vi "10 Balls.vi"() -> ()   [LabVIEW 2019]
uses:
  Team Code/TurretMode.ctl
  Team Code/MotorsGlobal.vi
  Team Code/JoysticksGlobal.vi
  Default10BallEnum.ctl
panel:
  in  "Delay After CurvaDir3":i32
  in  "RangeCurvaDir3":cluster{"output high":dbl, "output low":dbl}={"output high"=0.6, "output low"=-0.6} {"output low" format="%.2f"; "output high" format="%.2f"}
  in  "GainsCurvaDir3":T1={"proportional gain (Kc)"=1.0, "integral time (Ti, min)"=0.01, "derivative time (Td, min)"=0.0} {"derivative time (Td, min)" format="%.3f"; "integral time (Ti, min)" format="%.3f"; "proportional gain (Kc)" format="%.3f"}
  in  "Setpoint_CurvaDir3":dbl
  in  "TimeLimit_CurvaDir3":dbl
  in  "Delay After CurvaEsq2":i32
  in  "Delay After CurvaEsq1":i32
  in  "TimeLimit_Anda2":dbl
  in  "DelayAnda2":i32=300
  in  "Distance2":dbl
  in  "PID 10 Ball":T2(tab)
  in  "Distance1":dbl
  in  "DelayAnda1":i32=300
  in  "TimeLimit_Anda1":dbl
  in  "GainsCurvaEsq1":T1={"proportional gain (Kc)"=1.0, "integral time (Ti, min)"=0.01, "derivative time (Td, min)"=0.0} {"derivative time (Td, min)" format="%.3f"; "integral time (Ti, min)" format="%.3f"; "proportional gain (Kc)" format="%.3f"}
  in  "RangeCurvaEsq1":cluster{"output high":dbl, "output low":dbl}={"output high"=0.6, "output low"=-0.6} {"output low" format="%.2f"; "output high" format="%.2f"}
  in  "TimeLimit_CurvaEsq1":dbl
  in  "Setpoint_CurvaEsq1":dbl
  in  "Distance2":dbl
  in  "DelayAnda2":i32=300
  in  "TimeLimit_Anda2":dbl
  in  "GainsCurvaEsq2":T1={"proportional gain (Kc)"=1.0, "integral time (Ti, min)"=0.01, "derivative time (Td, min)"=0.0} {"derivative time (Td, min)" format="%.3f"; "integral time (Ti, min)" format="%.3f"; "proportional gain (Kc)" format="%.3f"}
  in  "RangeCurvaEsq2":cluster{"output high":dbl, "output low":dbl}={"output high"=0.6, "output low"=-0.6} {"output low" format="%.2f"; "output high" format="%.2f"}
  in  "TimeLimit_CurvaEsq2":dbl
  in  "Setpoint_CurvaEsq2":dbl
  in  "TimeLimit_AlinhaLL1":dbl
  in  "TimeLimit_Atira1":dbl
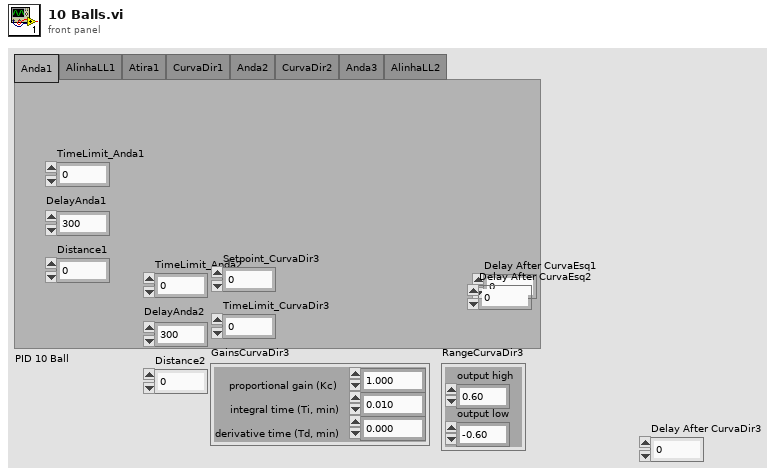
[diagram p1: front panel]
types:
  T1 = cluster{"proportional gain (Kc)":dbl, "integral time (Ti, min)":dbl, "derivative time (Td, min)":dbl}
  T2 = enum32{"Anda1", "AlinhaLL1", "Atira1", "CurvaDir1", "Anda2", "CurvaDir2", "Anda3", "AlinhaLL2"}
  T3 = typedef "Default10BallEnum.ctl" = enum16{"Reset1", "Anda1", "Reset2", "AndaAtras2", "CurvaEsq1", "Reset3", "Anda3", "CurvaEsq2", "Reset4", "AlinhaLL1", "Atira1", "CurvaDir3", "Reset5", "Anda4", "CurvaDir4", "Reset6", "Anda5", "AlinhaLL2", "Atira2"}
  T4 = typedef "TurretMode.ctl" = enum16{"Static", "Manual", "Automatic"}
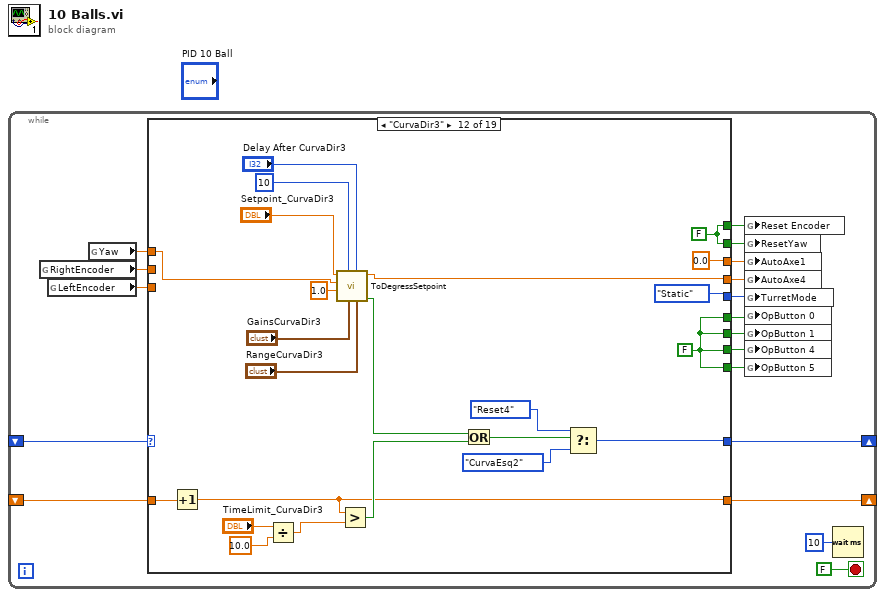
[diagram p0: block diagram]
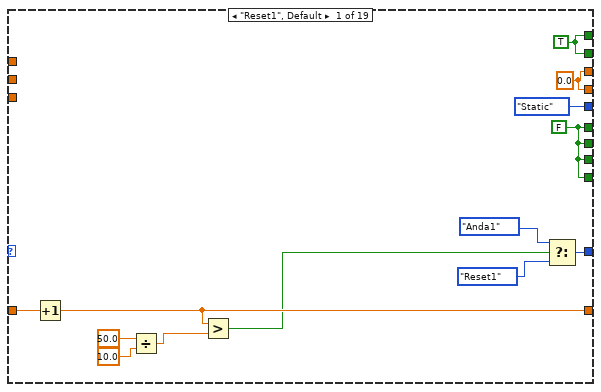
[diagram p2: hidden frame]
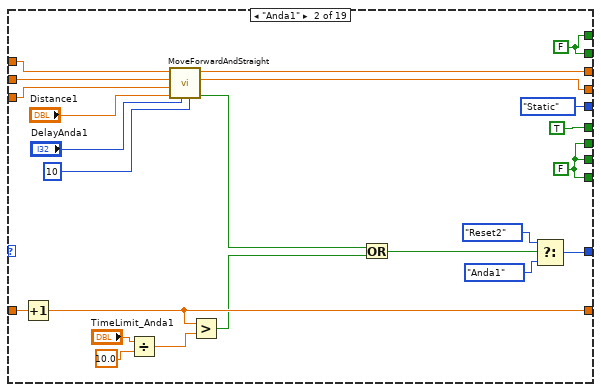
[diagram p3: hidden frame]
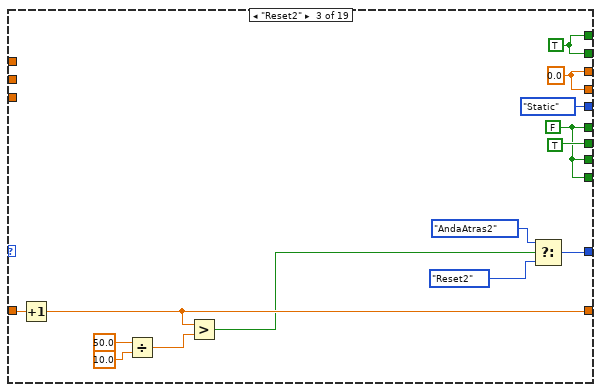
[diagram p4: hidden frame]
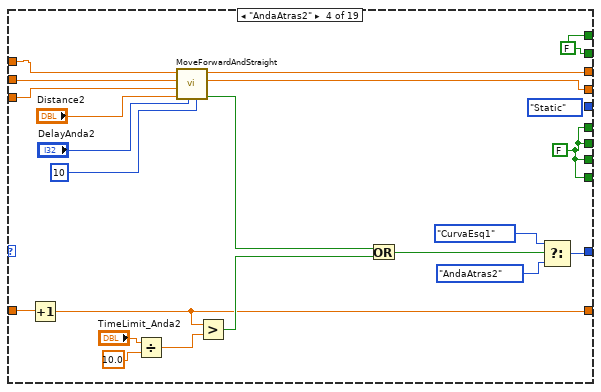
[diagram p5: hidden frame]
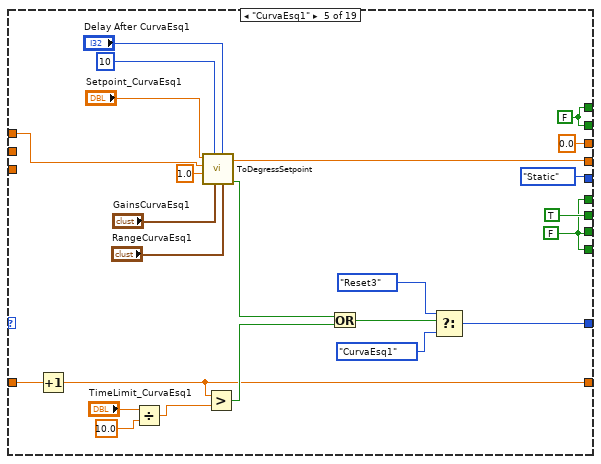
[diagram p6: hidden frame]
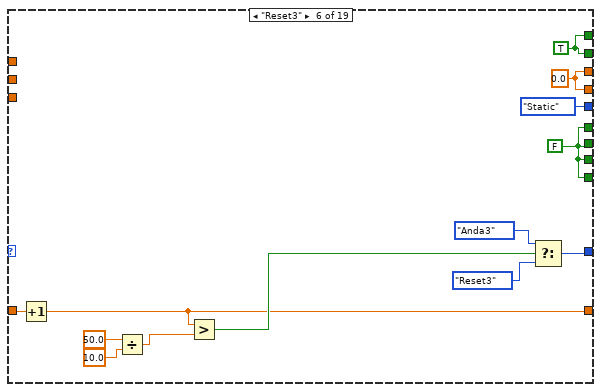
[diagram p7: hidden frame]
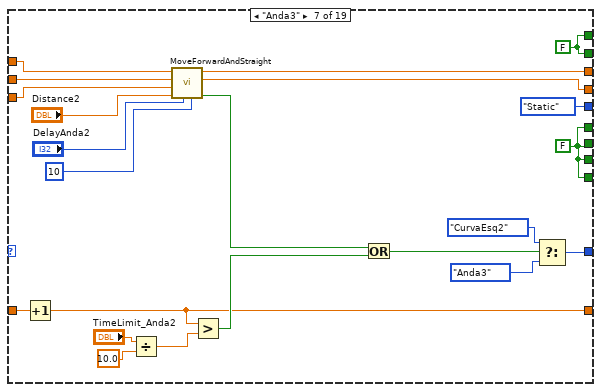
[diagram p8: hidden frame]
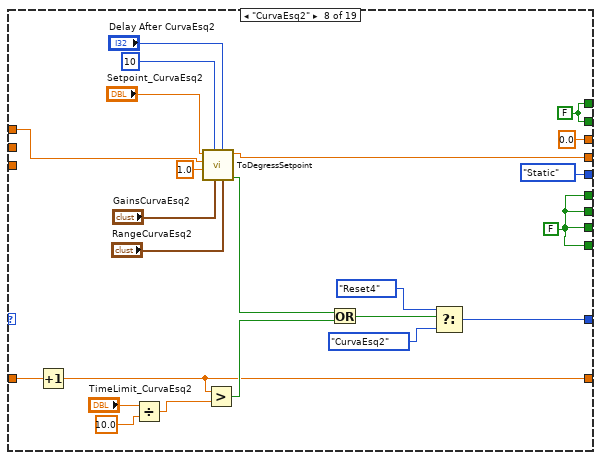
[diagram p9: hidden frame]
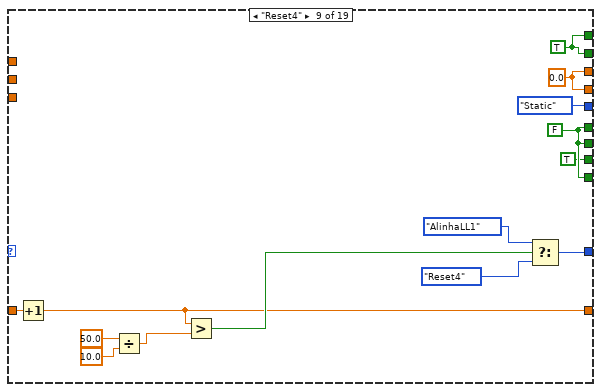
[diagram p10: hidden frame]
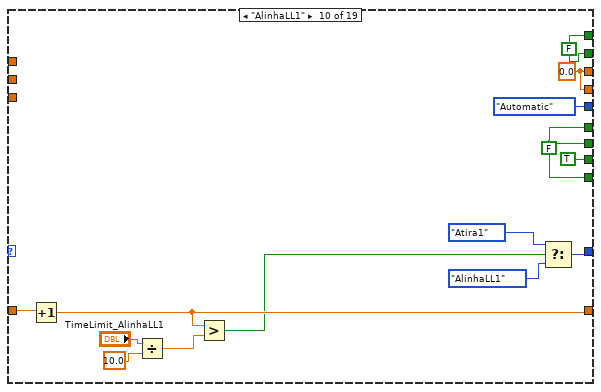
[diagram p11: hidden frame]
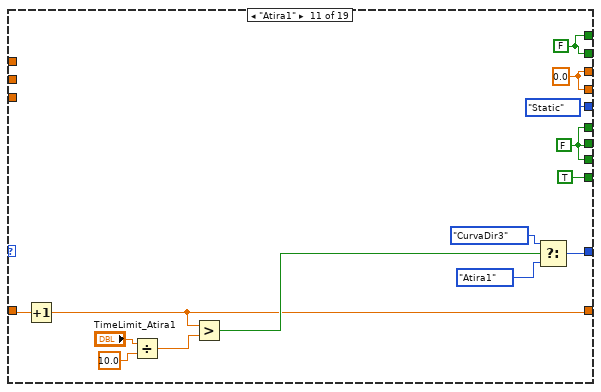
[diagram p12: hidden frame]
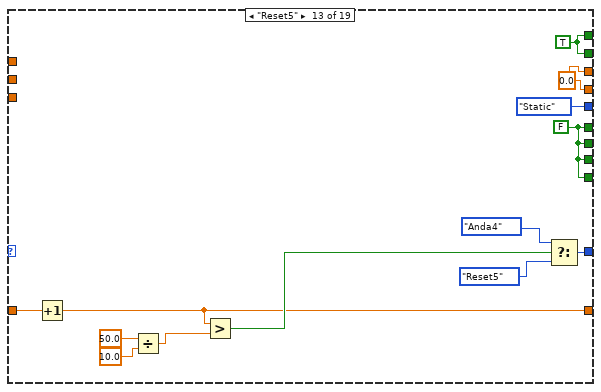
[diagram p13: hidden frame]
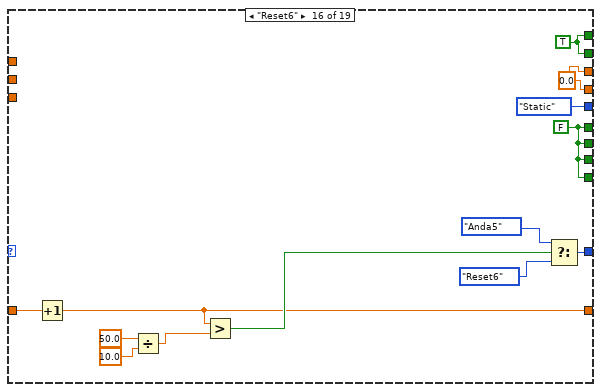
[diagram p16: hidden frame]
diagram:
  n1 = while {
    shift-right: [w15] -> _
    shift-left: _ -> [w16]
    shift-right: [w1] -> _
    shift-left: _ -> [w2]
    stop <- FALSE stop-if-true
    n2 = global read "MotorsGlobal.vi" "RightEncoder"() -> (w13:dbl)
    n3 = global read "MotorsGlobal.vi" "LeftEncoder"() -> (w12:dbl)
    n4 = global read "MotorsGlobal.vi" "Yaw"() -> (w14:dbl)
    n5 = case shown="\"CurvaDir3\"" w16 {
      tunnel: [w31 w46 w61 w76 w103 w116 w137 w159 w179 w191 w208 w218 w241 _ _ w252 _ _ _] -> w15
      tunnel: w14 -> [_ w49 _ w73 w102 _ w134 w162 _ _ _ w220 _ _ _ _ _ _ _]
      tunnel: w13 -> [_ w48 _ w72 _ _ w133 _ _ _ _ _ _ _ _ _ _ _ _]
      tunnel: w12 -> [_ w47 _ w71 _ _ w132 _ _ _ _ _ _ _ _ _ _ _ _]
      tunnel: [w30 w37 w66 w70 w100 w126 w135 w156 w181 w196 w209 w214 w238 _ _ w256 _ _ _] -> w11
      tunnel: [w30 w37 w66 w70 w100 w126 w135 w156 w181 w196 w209 w214 w238 _ _ w256 _ _ _] -> w10
      tunnel: [w29 w51 w67 w74 0.0 ("Trottle") w125 w130 0.0 ("Trottle") w177 w189 w204 0.0 ("Trottle") w237 _ _ w253 _ _ _] -> w9
      tunnel: [w29 w50 w67 w75 w99 w125 w131 w158 w177 w189 w204 w219 w237 _ _ w253 _ _ _] -> w8
      tunnel: [TurretMode."Static" ("TurretMode") TurretMode."Static" ("TurretMode") TurretMode."Static" ("TurretMode") _ TurretMode."Static" ("TurretMode") TurretMode."Static" ("TurretMode") TurretMode."Static" ("TurretMode") TurretMode."Static" ("TurretMode") TurretMode."Static" ("TurretMode") TurretMode."Automatic" ("TurretMode") TurretMode."Static" ("TurretMode") TurretMode."Static" ("TurretMode") TurretMode."Static" ("TurretMode") _ _ TurretMode."Static" ("TurretMode") _ _ _] -> w7
      tunnel: [w27 TRUE ("OpButton 0") w55 w69 w97 w123 w136 w149 w178 w195 w202 w216 w239 _ _ w255 _ _ _] -> w6
      tunnel: [w27 w36 w55 w69 w97 w123 w136 w149 w178 w195 TRUE w216 w239 _ _ w255 _ _ _] -> w5
      tunnel: [w27 w36 w55 w69 w97 w123 w136 w149 TRUE ("OpButton 0") TRUE ("OpButton 0") w202 w216 w239 _ _ w255 _ _ _] -> w4
      tunnel: [w27 w36 TRUE ("OpButton 0") w69 TRUE w123 w136 w149 w178 w195 w202 w216 w239 _ _ w255 _ _ _] -> w3
      tunnel: w2 -> [w24 w40 w63 w78 w95 w118 w139 w161 w175 w193 w207 w222 w243 _ _ w250 _ _ _]
      tunnel: [w23 w39 w62 w77 w94 w117 w138 w160 w180 w192 w206 w221 w242 _ _ w251 _ _ _] -> w1
      frame "Reset1", Default {
        w27 = FALSE ("OpButton 0")
        w29 = 0.0
        w30 = TRUE
        n6 = Increment(x=w24) -> (x+1=w23:dbl)
        n7 = Divide(x=50.0, y=10.0) -> (x/y=w25:dbl)
        n8 = Greater?(x=w23, y=w25) -> (0:w21:bool)
        n9 = Select(t=Default10BallEnum."Anda1", s=w21, f=Default10BallEnum."Reset1") -> (s? t:f=w31:T3)
      }
      frame "Anda1" {
        w37 = FALSE
        w36 = FALSE
        n10 = Increment(x=w40) -> (x+1=w39:dbl)
        n11 = Divide(x="TimeLimit_Anda1", y=10.0) -> (x/y=w42:dbl)
        n12 = call "MoveForwardAndStraight.vi"("Loop Timer"=10, "Time to stop"="DelayAnda1", "Distance"="Distance1", "Encoder Left"=w47, "Encoder Right"=w48, "Yaw"=w49) -> ("Finished distance"=w44:bool, "Direction"=w50:dbl, "Trottle"=w51:dbl)  [unwired: 2 in, 1 out]
        n13 = Greater?(x=w39, y=w42) -> (0:w38:bool)
        n14 = Or(x=w44, y=w38) -> (x .or. y?=w45:bool)
        n15 = Select(t=Default10BallEnum."Reset2", s=w45, f=Default10BallEnum."Anda1") -> (s? t:f=w46:T3)
      }
      frame "Reset2" {
        w66 = TRUE
        w67 = 0.0
        w55 = FALSE
        n16 = Increment(x=w63) -> (x+1=w62:dbl)
        n17 = Divide(x=50.0, y=10.0) -> (x/y=w65:dbl)
        n18 = Greater?(x=w62, y=w65) -> (0:w60:bool)
        n19 = Select(t=Default10BallEnum."AndaAtras2", s=w60, f=Default10BallEnum."Reset2") -> (s? t:f=w61:T3)
      }
      frame "AndaAtras2" {
        (unwired) TurretMode."Static" ("TurretMode")
        w70 = FALSE
        w69 = FALSE
        n20 = Increment(x=w78) -> (x+1=w77:dbl)
        n21 = Divide(x="TimeLimit_Anda2", y=10.0) -> (x/y=w83:dbl)
        n22 = call "MoveForwardAndStraight.vi"("Loop Timer"=10, "Time to stop"="DelayAnda2", "Distance"="Distance2", "Encoder Left"=w71, "Encoder Right"=w72, "Yaw"=w73) -> ("Finished distance"=w85:bool, "Direction"=w75:dbl, "Trottle"=w74:dbl)  [unwired: 2 in, 1 out]
        n23 = Greater?(x=w77, y=w83) -> (0:w81:bool)
        n24 = Or(x=w85, y=w81) -> (x .or. y?=w86:bool)
        n25 = Select(t=Default10BallEnum."CurvaEsq1", s=w86, f=Default10BallEnum."AndaAtras2") -> (s? t:f=w76:T3)
      }
      frame "CurvaEsq1" {
        w97 = FALSE
        w100 = FALSE
        n26 = Increment(x=w95) -> (x+1=w94:dbl)
        n27 = Divide(x="TimeLimit_CurvaEsq1", y=10.0) -> (x/y=w111:dbl)
        n28 = call "ToDegressSetpoint.vi"("Range"="RangeCurvaEsq1", "Delay After"="Delay After CurvaEsq1", "Gains"="GainsCurvaEsq1", "Loop Wait Delay"=10, "Precision"=1.0, "Yaw"=w102, "Setpoint (degress)"="Setpoint_CurvaEsq1") -> ("Finished?"=w104:bool, "Output"=w99:dbl)  [unwired: 3 in]
        n29 = Greater?(x=w94, y=w111) -> (0:w105:bool)
        n30 = Or(x=w104, y=w105) -> (x .or. y?=w106:bool)
        n31 = Select(t=Default10BallEnum."Reset3", s=w106, f=Default10BallEnum."CurvaEsq1") -> (s? t:f=w103:T3)
      }
      frame "Reset3" {
        w123 = FALSE
        w125 = 0.0
        w126 = TRUE
        n32 = Increment(x=w118) -> (x+1=w117:dbl)
        n33 = Divide(x=50.0, y=10.0) -> (x/y=w121:dbl)
        n34 = Greater?(x=w117, y=w121) -> (0:w119:bool)
        n35 = Select(t=Default10BallEnum."Anda3", s=w119, f=Default10BallEnum."Reset3") -> (s? t:f=w116:T3)
      }
      frame "Anda3" {
        w135 = FALSE
        w136 = FALSE
        n36 = Increment(x=w139) -> (x+1=w138:dbl)
        n37 = Divide(x="TimeLimit_Anda2", y=10.0) -> (x/y=w142:dbl)
        n38 = call "MoveForwardAndStraight.vi"("Loop Timer"=10, "Time to stop"="DelayAnda2", "Distance"="Distance2", "Encoder Left"=w132, "Encoder Right"=w133, "Yaw"=w134) -> ("Finished distance"=w144:bool, "Direction"=w131:dbl, "Trottle"=w130:dbl)  [unwired: 2 in, 1 out]
        n39 = Greater?(x=w138, y=w142) -> (0:w140:bool)
        n40 = Or(x=w144, y=w140) -> (x .or. y?=w145:bool)
        n41 = Select(t=Default10BallEnum."CurvaEsq2", s=w145, f=Default10BallEnum."Anda3") -> (s? t:f=w137:T3)
      }
      frame "CurvaEsq2" {
        w149 = FALSE
        w156 = FALSE
        n42 = Increment(x=w161) -> (x+1=w160:dbl)
        n43 = Divide(x="TimeLimit_CurvaEsq2", y=10.0) -> (x/y=w169:dbl)
        n44 = call "ToDegressSetpoint.vi"("Range"="RangeCurvaEsq2", "Delay After"="Delay After CurvaEsq2", "Gains"="GainsCurvaEsq2", "Loop Wait Delay"=10, "Precision"=1.0, "Yaw"=w162, "Setpoint (degress)"="Setpoint_CurvaEsq2") -> ("Finished?"=w163:bool, "Output"=w158:dbl)  [unwired: 3 in]
        n45 = Greater?(x=w160, y=w169) -> (0:w164:bool)
        n46 = Or(x=w163, y=w164) -> (x .or. y?=w154:bool)
        n47 = Select(t=Default10BallEnum."Reset4", s=w154, f=Default10BallEnum."CurvaEsq2") -> (s? t:f=w159:T3)
      }
      frame "Reset4" {
        w178 = FALSE
        w177 = 0.0
        w181 = TRUE
        n48 = Increment(x=w175) -> (x+1=w180:dbl)
        n49 = Divide(x=50.0, y=10.0) -> (x/y=w184:dbl)
        n50 = Greater?(x=w180, y=w184) -> (0:w182:bool)
        n51 = Select(t=Default10BallEnum."AlinhaLL1", s=w182, f=Default10BallEnum."Reset4") -> (s? t:f=w179:T3)
      }
      frame "AlinhaLL1" {
        w189 = 0.0 ("Trottle")
        w196 = FALSE
        w195 = FALSE
        n52 = Increment(x=w193) -> (x+1=w192:dbl)
        n53 = Divide(x="TimeLimit_AlinhaLL1", y=10.0) -> (x/y=w198:dbl)
        n54 = Greater?(x=w192, y=w198) -> (0:w190:bool)
        n55 = Select(t=Default10BallEnum."Atira1", s=w190, f=Default10BallEnum."AlinhaLL1") -> (s? t:f=w191:T3)
      }
      frame "Atira1" {
        w209 = FALSE
        w204 = 0.0
        w202 = FALSE
        n56 = Increment(x=w207) -> (x+1=w206:dbl)
        n57 = Divide(x="TimeLimit_Atira1", y=10.0) -> (x/y=w212:dbl)
        n58 = Greater?(x=w206, y=w212) -> (0:w210:bool)
        n59 = Select(t=Default10BallEnum."CurvaDir3", s=w210, f=Default10BallEnum."Atira1") -> (s? t:f=w208:T3)
      }
      frame "CurvaDir3" {
        w216 = FALSE
        w214 = FALSE
        n60 = Increment(x=w222) -> (x+1=w221:dbl)
        n61 = Divide(x="TimeLimit_CurvaDir3", y=10.0) -> (x/y=w234:dbl)
        n62 = call "ToDegressSetpoint.vi"("Range"="RangeCurvaDir3", "Delay After"="Delay After CurvaDir3", "Gains"="GainsCurvaDir3", "Loop Wait Delay"=10, "Precision"=1.0, "Yaw"=w220, "Setpoint (degress)"="Setpoint_CurvaDir3") -> ("Finished?"=w228:bool, "Output"=w219:dbl)  [unwired: 3 in]
        n63 = Greater?(x=w221, y=w234) -> (0:w229:bool)
        n64 = Or(x=w228, y=w229) -> (x .or. y?=w227:bool)
        n65 = Select(t=Default10BallEnum."Reset4", s=w227, f=Default10BallEnum."CurvaEsq2") -> (s? t:f=w218:T3)
      }
      frame "Reset5" {
        w239 = FALSE ("OpButton 0")
        w237 = 0.0
        w238 = TRUE
        n66 = Increment(x=w243) -> (x+1=w242:dbl)
        n67 = Divide(x=50.0, y=10.0) -> (x/y=w248:dbl)
        n68 = Greater?(x=w242, y=w248) -> (0:w246:bool)
        n69 = Select(t=Default10BallEnum."Anda4", s=w246, f=Default10BallEnum."Reset5") -> (s? t:f=w241:T3)
      }
      frame "Anda4" {
      }
      frame "CurvaDir4" {
      }
      frame "Reset6" {
        w255 = FALSE ("OpButton 0")
        w253 = 0.0
        w256 = TRUE
        n70 = Increment(x=w250) -> (x+1=w251:dbl)
        n71 = Divide(x=50.0, y=10.0) -> (x/y=w261:dbl)
        n72 = Greater?(x=w251, y=w261) -> (0:w259:bool)
        n73 = Select(t=Default10BallEnum."Anda5", s=w259, f=Default10BallEnum."Reset6") -> (s? t:f=w252:T3)
      }
      frame "Anda5" {
      }
      frame "AlinhaLL2" {
      }
      frame "Atira2" {
      }
    }
    n74 = global write "MotorsGlobal.vi" "Reset Encoder"(w11) -> ()
    n75 = global write "MotorsGlobal.vi" "ResetYaw"(w10) -> ()
    n76 = global write "JoysticksGlobal.vi" "AutoAxe1"(w9) -> ()
    n77 = global write "JoysticksGlobal.vi" "AutoAxe4"(w8) -> ()
    n78 = global write "MotorsGlobal.vi" "TurretMode"(w7) -> ()
    n79 = global write "JoysticksGlobal.vi" "OpButton 0"(w6) -> ()
    n80 = global write "JoysticksGlobal.vi" "OpButton 1"(w3) -> ()
    n81 = global write "JoysticksGlobal.vi" "OpButton 4"(w4) -> ()
    n82 = global write "JoysticksGlobal.vi" "OpButton 5"(w5) -> ()
    n83 = Wait (ms)(milliseconds to wait=u32 10) -> ()  [unwired: 1 out]
  }
